vi "LM35 INTERFACING USING DAQ CARD.vi"() -> ()   [LabVIEW 2021]
uses:
  <vilib>/DAQmx/read.llb/DAQmx Read (Analog DBL 1Chan 1Samp).vi
  <vilib>/DAQmx/create/channels.llb/DAQmx Create Channel (AI-Voltage-Basic).vi
  <vilib>/DAQmx/miscellaneous.llb/DAQmx Fill In Error Info.vi
panel:
  in  "stop":bool
  out "TEMPERATURE":dbl
  out "Waveform Chart":dbl(graph)
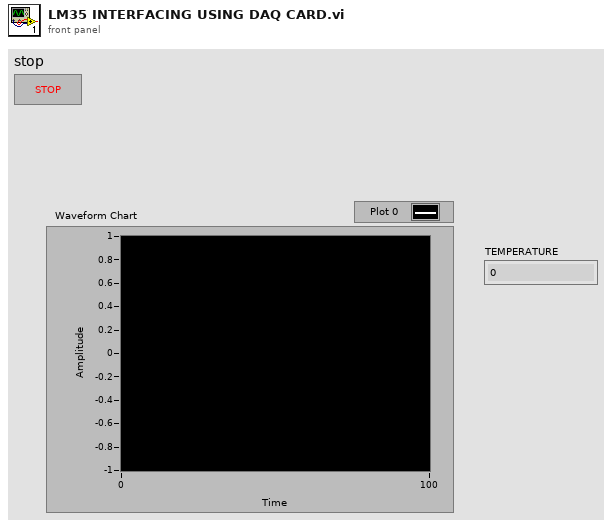
[diagram p1: front panel]
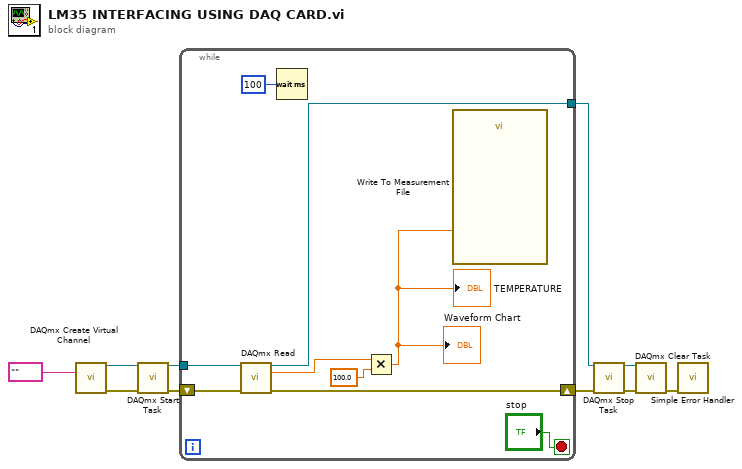
[diagram p0: block diagram]
diagram:
  n1 = call-poly <vilib>:"DAQmx Create Virtual Channel.vi"("physical channels"=tag "") -> ("task out"=w9:refnum<k21>, "error out"=w8:errorcluster)  [unwired: 13 in]
  n2 = call <vilib>:"DAQmx Start Task.vi"("task/channels in"=w9, "error in"=w8) -> ("task out"=w2:refnum<k21>, "error out"=w7:errorcluster)  [unwired: 12 in]
  n3 = while {
    shift-right: [w18] -> w6
    shift-left: w7 -> [w19]
    tunnel: w2 -> [w14]
    tunnel: [w13] -> w1
    stop <- "stop" stop-if-true
    n4 = call-poly <vilib>:"DAQmx Read.vi"("task/channels in"=w14, "error in"=w19) -> ("task out"=w13:refnum<k21>, "data"=w16:dbl, "error out"=w18:errorcluster)  [unwired: 11 in]
    n5 = Wait (ms)(milliseconds to wait=u32 100) -> ()  [unwired: 1 out]
    n6 = Multiply(x=w16, y=100.0) -> (x*y=w12:dbl)
    "TEMPERATURE" <- w12
    "Waveform Chart" <- w12
    n7 = call "Write To Measurement File"("Signals"=w12) -> ()  [unwired: 16 in, 3 out]
  }
  n8 = call <vilib>:"DAQmx Stop Task.vi"("task/channels in"=w1, "error in"=w6) -> ("task out"=w4:refnum<k21>, "error out"=w5:errorcluster)  [unwired: 12 in]
  n9 = call <vilib>:"DAQmx Clear Task.vi"("task in"=w4, "error in"=w5) -> ("error out"=w10:errorcluster)  [unwired: 13 in]
  n10 = call <vilib>:"Simple Error Handler.vi"("error in (no error)"=w10) -> ()  [unwired: 4 in, 5 out]
